vi "Process.vi"(8 "error in (no error)":errorcluster, 11 "Error Handler In":refnum<class "Error Handler.lvclass">) -> (0 "error out":errorcluster, 3 "Error Handler Out":refnum<class "Error Handler.lvclass">)   [LabVIEW 2020, in "Error Handler.lvclass"]
uses:
  Error Handler.lvclass
  C:/Git/astemes-lunit/source/Application Framework/Process Classes/Process/Process.lvclass
  Error Handler.lvclass/Error Handler.ctl
  Process/Process.lvclass/Process.ctl
  Public/TypeDefs/Error Message Data.ctl
  <vilib>/Utility/error.llb/Error Cluster From Error Code.vi
  Support/Error Log Classes/Error Log/Error Log.lvclass
  Process/Process.lvclass
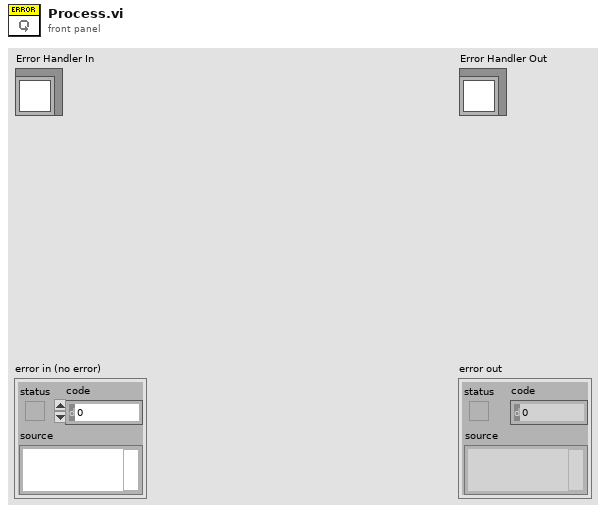
[diagram p1: front panel]
types:
  T1 = typedef "Error Handler.lvclass/Error Message Data.ctl" = cluster{"Error Type":string, "Location":string, "Error":errorcluster}
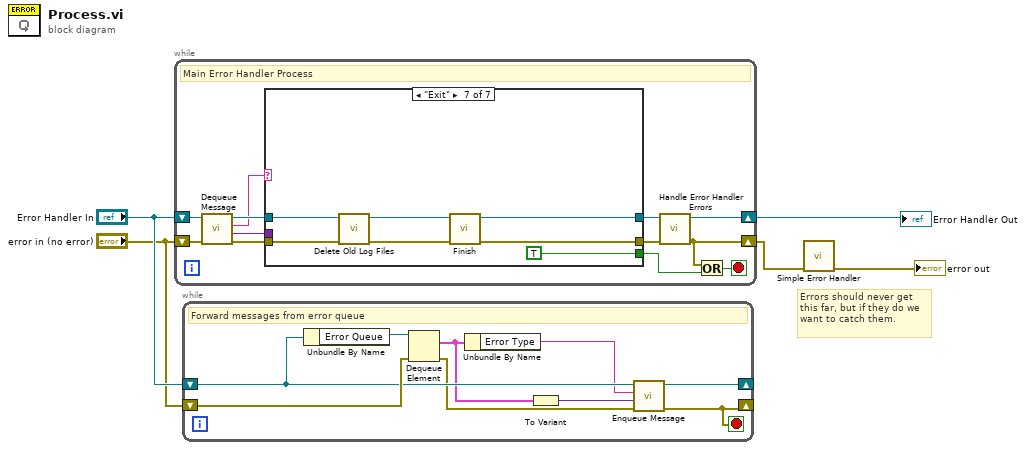
[diagram p0: block diagram]
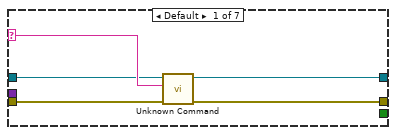
[diagram p2: hidden frame]
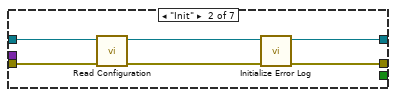
[diagram p3: hidden frame]
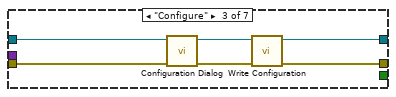
[diagram p4: hidden frame]
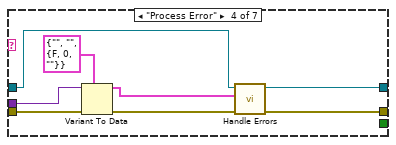
[diagram p5: hidden frame]
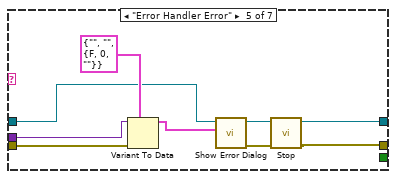
[diagram p6: hidden frame]
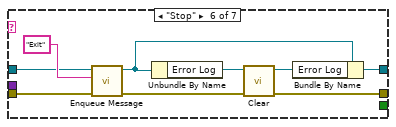
[diagram p7: hidden frame]
diagram:
  # "Errors should never get this far, but if they do we want to catch them."
  n1 = while {
    shift-right: [w7] -> w2
    shift-left: "error in (no error)" -> [w16]
    shift-right: [w10] -> w5
    shift-left: "Error Handler In" -> [w17]
    stop <- w8 stop-if-true
    # "Main Error Handler Process"
    n2 = call "Dequeue Message.vi"("error in (no error)"=w16, "Process In"=w17) -> ("error out"=w15:errorcluster, "Message Data"=w12:variant, "Message"=w13:string, "Process Out"=w14:refnum<class "Error Handler.lvclass">)  [unwired: 6 in]
    n3 = case shown="\"Exit\"" w13 {
      selector: w13 -> [w22 _ _ _ _ _ _]
      tunnel: [w19 w25 w30 w36 w47 w52 w65] -> w9
      tunnel: w15 -> [w18 w27 w33 w40 w51 w58 w63]
      tunnel: [w21 w23 w29 w35 w49 w55 w66] -> w6
      tunnel: w14 -> [w20 w28 w34 w38 w45 w59 w61]
      tunnel: w12 -> [_ _ _ w42 w50 _ _]
      tunnel: [_ _ _ _ _ _ TRUE] -> w11
      frame Default {
        n4 = call "Unknown Command.vi"("error in (no error)"=w18, "String"=w22, "Process In"=w20) -> ("error out"=w19:errorcluster, "Process Out"=w21:refnum<class "Error Handler.lvclass">)  [unwired: 7 in]
      }
      frame "Init" {
        n5 = call-dynamic "Read Configuration.vi"("error in (no error)"=w27, "Error Handler In"=w28) -> ("error out"=w26:errorcluster, "Error Handler Out"=w24:refnum<class "Error Handler.lvclass">)  [unwired: 8 in]
        n6 = call "Initialize Error Log.vi"("error in (no error)"=w26, "Error Handler In"=w24) -> ("error out"=w25:errorcluster, "Error Handler Out"=w23:refnum<class "Error Handler.lvclass">)  [unwired: 8 in]
      }
      frame "Configure" {
        n7 = call "Configuration Dialog.vi"("error in (no error)"=w33, "Error Handler In"=w34) -> ("error out"=w31:errorcluster, "Error Handler Out"=w32:refnum<class "Error Handler.lvclass">)  [unwired: 8 in]
        n8 = call-dynamic "Write Configuration.vi"("error in (no error)"=w31, "Error Handler In"=w32) -> ("error out"=w30:errorcluster, "Error Handler Out"=w29:refnum<class "Error Handler.lvclass">)  [unwired: 8 in]
      }
      frame "Process Error" {
        n9 = Variant To Data(error in=w40, type=T1 {"Error Type"="", "Location"="", "Error"={"status"=FALSE, "code"=0, "source"=""}} ("Error Message Data"), Variant=w42) -> (data=w39:T1, error out=w37:errorcluster)
        n10 = call "Handle Errors.vi"("error in (no error)"=w37, "Error Message Data"=w39, "Error Handler In"=w38) -> ("error out"=w36:errorcluster, "Error Handler Out"=w35:refnum<class "Error Handler.lvclass">)  [unwired: 7 in]
      }
      frame "Error Handler Error" {
        n11 = Variant To Data(error in=w51, type=T1 {"Error Type"="", "Location"="", "Error"={"status"=FALSE, "code"=0, "source"=""}} ("Error Message Data"), Variant=w50) -> (data=w44:T1)  [unwired: 1 out]
        n12 = call "Show Error Dialog.vi"("Error Message Data"=w44, "Error Handler In"=w45) -> ("error out"=w43:errorcluster, "Error Handler Out"=w46:refnum<class "Error Handler.lvclass">)  [unwired: 8 in]
        n13 = call-dynamic "Stop.vi"("error in (no error)"=w43, "Process In"=w46) -> ("error out"=w47:errorcluster, "Process Out"=w49:refnum<class "Error Handler.lvclass">)  [unwired: 7 in, 1 out]
      }
      frame "Stop" {
        n14 = call "Enqueue Message.vi"("error in (no error)"=w58, "Message"="Exit", "Process In"=w59) -> ("error out"=w53:errorcluster, "Process Out"=w57:refnum<class "Error Handler.lvclass">)  [unwired: 7 in]
        n15 = Unbundle By Name(w57) -> ("Error Log"=w56:refnum<class "Error Log.lvclass">)
        n16 = call-dynamic "Clear.vi"("error in (no error)"=w53, "Error Log in"=w56) -> ("error out"=w52:errorcluster, "Error Log out"=w54:refnum<class "Error Log.lvclass">)  [unwired: 7 in, 1 out]
        n17 = Bundle By Name(cluster=w57, "Error Log"=w54) -> (w55:refnum<class "Error Handler.lvclass">)
      }
      frame "Exit" {
        n18 = call "Delete Old Log Files.vi"("error in (no error)"=w63, "Error Handler In"=w61) -> ("error out"=w64:errorcluster, "Error Handler Out"=w62:refnum<class "Error Handler.lvclass">)  [unwired: 8 in]
        n19 = call "Finish.vi"("error in (no error)"=w64, "Process In"=w62) -> ("error out"=w65:errorcluster, "Process Out"=w66:refnum<class "Error Handler.lvclass">)  [unwired: 8 in]
      }
    }
    n20 = call "Handle Error Handler Errors.vi"("error in (no error)"=w9, "Process In"=w6) -> ("error out"=w7:errorcluster, "Process Out"=w10:refnum<class "Error Handler.lvclass">)  [unwired: 8 in]
    n21 = Or(x=w7, y=w11) -> (x .or. y?=w8:bool)
  }
  "Error Handler Out" <- w5
  n22 = while {
    shift-right: [w68] -> _
    shift-left: "error in (no error)" -> [w75]
    shift-right: [w69] -> _
    shift-left: "Error Handler In" -> [w74]
    stop <- w68 stop-if-true
    # "Forward messages from error queue"
    n23 = Unbundle By Name(w74) -> ("Error Queue"=w76:refnum<queue>)
    n24 = Dequeue Element(queue=w76, error in (no error)=w75) -> (element=w72:T1, error out=w71:errorcluster)  [unwired: 1 in, 2 out]
    n25 = Unbundle By Name(w72) -> ("Error Type"=w73:string)
    n26 = To Variant(anything=w72) -> (Variant=w70:variant)
    n27 = call "Enqueue Message.vi"("error in (no error)"=w71, "Message Data"=w70, "Message"=w73, "Process In"=w74) -> ("error out"=w68:errorcluster, "Process Out"=w69:refnum<class "Error Handler.lvclass">)  [unwired: 6 in]
  }
  n28 = call <vilib>:"Simple Error Handler.vi"("error in (no error)"=w2) -> ("error out"=→"error out":errorcluster)  [unwired: 4 in, 4 out]
